vi "Untitled 1.vi"() -> ()   [LabVIEW 2010]
uses:
  <vilib>/NXT/Subs/MotorOutput.ctl
  <vilib>/NXT/Dual Mode Library/Motors/MotorOn.vi
  <vilib>/NXT/Dual Mode Library/Waits/Wait_Num.vi
  <vilib>/NXT/Dual Mode Library/Motors/MotorReverse.vi
  <vilib>/NXT/Dual Mode Library/Motors/MotorBrake.vi
panel:
  in  "Time (sec)":sgl=1.0
  in  "Output Port (All Ports)":T1=3 items=["Port A", "Port B", "Port C", "All Ports"]
  in  "Power (75)":i32=75
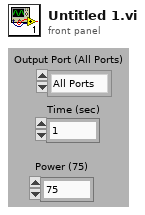
[diagram p1: front panel]
types:
  T1 = typedef "MotorOutput.ctl" = u8
  T2 = typedef "LVHSConnector.ctl" = cluster{"error":errorcluster, "address":string, "NXT #":i32, "Show Error":bool, "Connection":u16}
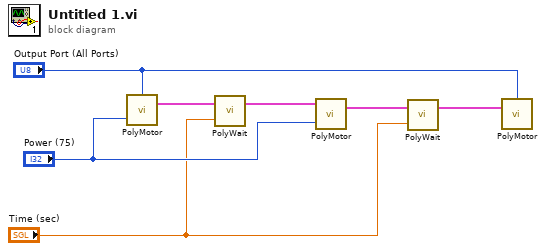
[diagram p0: block diagram]
diagram:
  n1 = call-poly <vilib>:"PolyMotor.vi"("Power (75)"="Power (75)", "Output Port (All Ports)"="Output Port (All Ports)") -> ("NXT"=w7:T2)  [unwired: 2 in]
  n2 = call-poly <vilib>:"PolyWait.vi"("Time (sec)"="Time (sec)", "NXT"=w7) -> ("NXT"=w6:T2)  [unwired: 2 in]
  n3 = call-poly <vilib>:"PolyMotor.vi"("Power (75)"="Power (75)", "NXT"=w6) -> ("NXT"=w5:T2)  [unwired: 2 in]
  n4 = call-poly <vilib>:"PolyWait.vi"("Time (sec)"="Time (sec)", "NXT"=w5) -> ("NXT"=w2:T2)  [unwired: 2 in]
  n5 = call-poly <vilib>:"PolyMotor.vi"("NXT"=w2, "Port (All Ports)"="Output Port (All Ports)") -> ()  [unwired: 2 in, 1 out]
